vi "Refresh Stats.vi"(11 "CIFCorePlugin in":refnum<class "CIFCorePlugin.lvclass">) -> (3 "CIFCorePlugin out":refnum<class "CIFCorePlugin.lvclass">)   [LabVIEW 2021, in "CIFCorePlugin.lvclass"]
uses:
  CIFCorePlugin.lvclass
  Common/Typedef/Timing Statistics.ctl
  Common/Typedef/Timing Stats Base.ctl
  Common/Typedef/FIFO Statistics.ctl
  Common/Typedef/Simple Error.ctl
  CIFCorePlugin.lvclass/CIFCorePlugin.ctl
  Common/CIFCoreCommon.lvlib
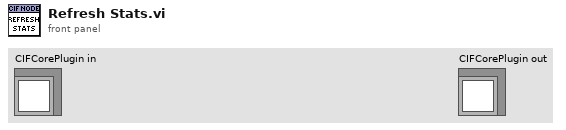
[diagram p1: front panel]
types:
  T1 = typedef "CIFCoreCommon.lvlib/Timing Statistics.ctl" = cluster{"Period":T2, "Wake Error":T2, "Execute":T2, "Housekeep":T2, "Idle":T2, "Cleanup":T2, "Custom 1 (custom units)":T2, "Custom 2 (custom units)":T2}
  T2 = typedef "CIFCoreCommon.lvlib/Timing Stats Base.ctl" = cluster{"Max":i64, "Avg":dbl, "Min":i64}
  T3 = typedef "CIFCoreCommon.lvlib/FIFO Statistics.ctl" = cluster{"From T0":T2, "From Previous Plugin":T2, "Output Error":T2}
  T4 = typedef "CIFCoreCommon.lvlib/Simple Error.ctl" = cluster{"status":bool, "code":i32}
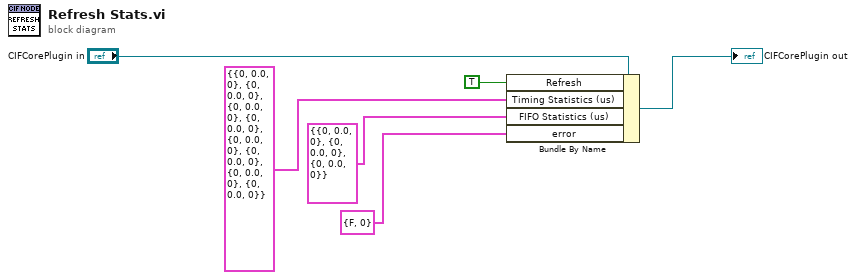
[diagram p0: block diagram]
diagram:
  n1 = Bundle By Name(cluster="CIFCorePlugin in", "Refresh"=TRUE, "Timing Statistics (us)"=T1 {"Period"={"Max"=0, "Avg"=0.0, "Min"=0}, "Wake Error"={"Max"=0, "Avg"=0.0, "Min"=0}, "Execute"={"Max"=0, "Avg"=0.0, "Min"=0}, "Housekeep"={"Max"=0, "Avg"=0.0, "Min"=0}, "Idle"={"Max"=0, "Avg"=0.0, "Min"=0}, "Cleanup"={"Max"=0, "Avg"=0.0, "Min"=0}, "Custom 1 (custom units)"={"Max"=0, "Avg"=0.0, "Min"=0}, "Custom 2 (custom units)"={"Max"=0, "Avg"=0.0, "Min"=0}} ("Status.Timing Statistics (us)"), "FIFO Statistics (us)"=T3 {"From T0"={"Max"=0, "Avg"=0.0, "Min"=0}, "From Previous Plugin"={"Max"=0, "Avg"=0.0, "Min"=0}, "Output Error"={"Max"=0, "Avg"=0.0, "Min"=0}} ("Status.FIFO Statistics (us)"), "error"=T4 {"status"=FALSE, "code"=0} ("Status.error")) -> (→"CIFCorePlugin out":refnum<class "CIFCorePlugin.lvclass">)
